vi "D3-latch.vi"(8 "CLK":bool, 11 "D":bool) -> (0 "'Q":bool, 3 "Q":bool)   [LabVIEW 2021]
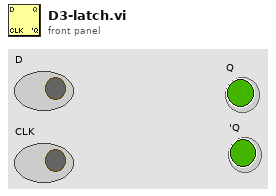
[diagram p1: front panel]
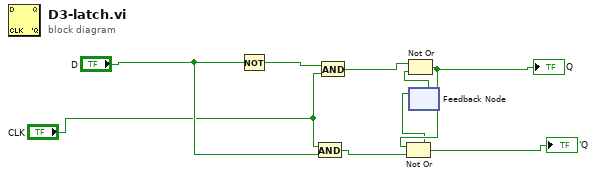
[diagram p0: block diagram]
diagram:
  n1 = Not(x="D") -> (.not. x?=w8:bool)
  n2 = And(x="CLK", y="D") -> (x .and. y?=w6:bool)
  n3 = And(x=w8, y="CLK") -> (x .and. y?=w7:bool)
  n4 = feedback #1() -> (w5:bool)  [unwired: 1 in]
  n5 = Not Or(1:w5, 2:w7) -> (0:w2:bool)
  "Q" <- w2
  n6 = Not Or(1:w6, 2:w2) -> (0:w1:bool)
  "'Q" <- w1
  n7 = feedback-in #1(w1) -> ()
